vi "T7_Write_DAC_Register.vi"(0 "Remote IP Address":string="192.168.126.148", 2 "FirstChannel":u16, 4 "FLOAT32 to Write":sgl=1.23) -> (9 "WrittenAt":timestamp=timestamp(3513857842.218402 s since 1904-01-01), 10 "error out":errorcluster)   [LabVIEW 2018]
panel:
  out "Starting Address":u16=1002
  # "MB Ethernet Example Master.vi\n\nInstructions\n1.Use Kipling to find your devices IP address & modify the\n\"Remote IP Addres\"\n2. Run this VI\n3. Change value of \"FLOAT32 to Write\" & press \"Write Data\""
  # "TCP Parameters"
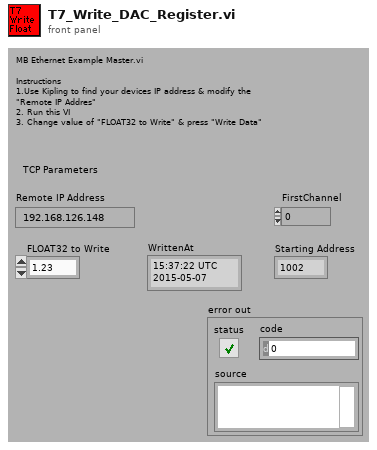
[diagram p1: front panel]
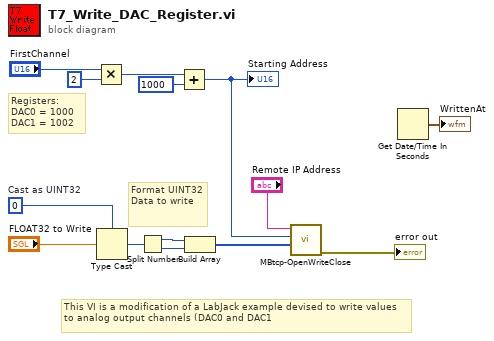
[diagram p0: block diagram]
diagram:
  w9 = u32 0  # Cast as UINT32
  # "This VI is a modification of a LabJack example devised to write values to analog output channels (DAC0 and DAC1"
  # "Format UINT32 Data to write"
  # "Registers:\nDAC0 = 1000\nDAC1 = 1002"
  n1 = Multiply(x="FirstChannel", y=u16 2) -> (x*y=w12:u16)
  n2 = Type Cast(type=w9, x="FLOAT32 to Write") -> (*(type *) &x=w8:u32)
  n3 = Split Number(x=w8) -> (hi(x)=w7:u16, lo(x)=w6:u16)
  n4 = Add(x=w12, y=u16 1000) -> (x+y=w3:u16)
  "Starting Address" <- w3
  n5 = Build Array(w7, w6) -> (w2:u16[])
  n6 = call "MBtcp-OpenWriteClose.vi"("Values"=w2, "RegisterAddr"=w3, "IP Address(:port)"="Remote IP Address") -> ("error out"=→"error out":errorcluster)  [unwired: 8 in]
  n7 = Get Date/Time In Seconds() -> (seconds since 1Jan1904=→"WrittenAt":timestamp)
